vi "Change File Extension.vi"(4 "New extension":string, 5 "File Path In":path) -> (1 "File Path Out":path)   [LabVIEW 2015]
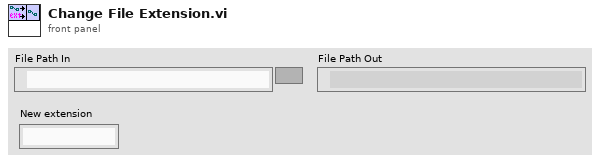
[diagram p1: front panel]
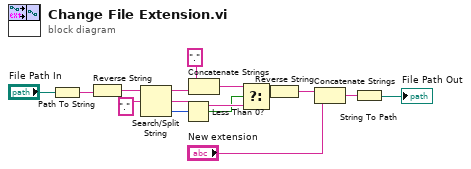
[diagram p0: block diagram]
diagram:
  n1 = Path To String(path="File Path In") -> (string=w9:string)
  n2 = Reverse String(1:w9) -> (0:w10:string)
  n3 = Search/Split String(string=w10, search string/char (-)=".") -> (substring before match=w2:string, match + rest of string=w6:string, offset of match=w7:i32)  [unwired: 1 in]
  n4 = Less Than 0?(x=w7) -> (x < 0?=w4:bool)
  n5 = Concatenate Strings("." ("string"), w2) -> (w1:string)
  n6 = Select(t=w1, s=w4, f=w6) -> (s? t:f=w5:string)
  n7 = Reverse String(1:w5) -> (0:w12:string)
  n8 = Concatenate Strings(w12, "New extension") -> (w13:string)
  n9 = String To Path(string=w13) -> (path=→"File Path Out":path)
